vi "Pressure Controller.vi"(7 "Set? (F:Read)":bool, 8 "Error In":errorcluster, 9 "Controller Code (STD)":enum16{"STD", "250", "152", "---", "652", "146"}(ring), 11 "VISA resource name":refnum<visa-resource-name>) -> (0 "Error Out":errorcluster, 1 "Controller Code out":enum16{"STD", "250", "152", "---", "652", "146"}(ring), 3 "dup VISA resource name":refnum<visa-resource-name>)   [LabVIEW 2011, in "MGC647C.lvlib"]
doc: "Read/set pressure controller."
uses:
  <instrlib>/MGC647C/MGC647C.lvlib
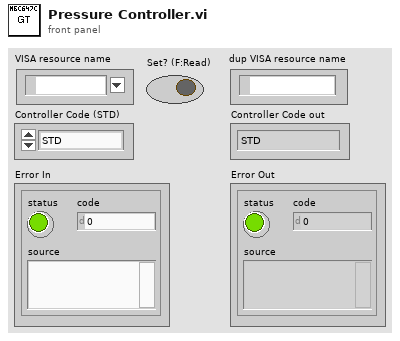
[diagram p1: front panel]
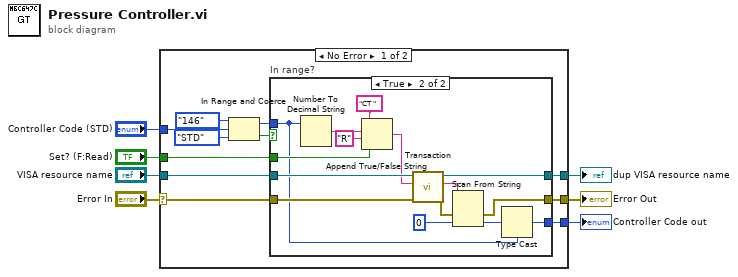
[diagram p0: block diagram]
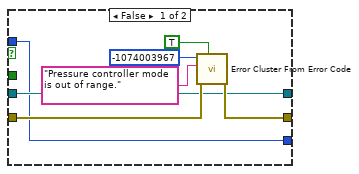
[diagram p2: hidden frame]
diagram:
  n1 = case shown="No Error" "Error In" {
    selector: "Error In" -> [w11 w42]
    tunnel: "VISA resource name" -> [w18 w41]
    tunnel: [w17 w41] -> w6
    tunnel: [w16 w42] -> w5
    tunnel: "Set? (F:Read)" -> [w15 _]
    tunnel: "Controller Code (STD)" -> [w14 w43]
    tunnel: [w10 w43] -> w1
    frame No Error {
      n2 = In Range and Coerce(upper limit=enum16{"STD", "250", "152", "---", "652", "146"}."146", x=w14, lower limit=enum16{"STD", "250", "152", "---", "652", "146"}."STD") -> (coerced(x)=w13:enum16{"STD", "250", "152", "---", "652", "146"}, In Range?=w12:bool)
      n3 = case "In range?" shown="True" w12 {
        tunnel: w18 -> [w23 w40]
        tunnel: [w23 w39] -> w17
        tunnel: [w24 w33] -> w16
        tunnel: w15 -> [_ w36]
        tunnel: w13 -> [w19 w27]
        tunnel: w11 -> [w25 w31]
        tunnel: [w19 w26] -> w10
        frame False {
          n4 = call <vilib>:"Error Cluster From Error Code.vi"("show call chain? (False)"=TRUE, "error in (no error)"=w25, "error message (\"\")"="Pressure controller mode is out of range." ("error message (\"\")"), "error code (0)"=-1074003967) -> ("error out"=w24:errorcluster)  [unwired: 5 in]
        }
        frame True {
          n5 = Number To Decimal String(number=w27) -> (decimal integer string=w30:string)  [unwired: 1 in]
          n6 = Append True/False String(1:w36, 2:"R" ("false string"), 3:w30, 4:"CT " ("string (\"\")")) -> (0:w32:string)
          n7 = call <instrlib>:"Transaction.vi"("Error In"=w31, "Command"=w32, "VISA resource name"=w40) -> ("Error Out"=w34:errorcluster, "Response"=w35:string, "dup VISA resource name"=w39:refnum<visa-resource-name>)  [unwired: 6 in]
          n8 = Scan From String(input string=w35, error in=w34, default 1=u16 0) -> (error out=w33:errorcluster, output 1=w28:u16)  [unwired: 2 in, 2 out]
          n9 = Type Cast(type=w27, x=w28) -> (*(type *) &x=w26:enum16{"STD", "250", "152", "---", "652", "146"})
        }
      }
    }
    frame Error {
    }
  }
  "dup VISA resource name" <- w6
  "Error Out" <- w5
  "Controller Code out" <- w1
